vi "Pointer producer consumer TDMS generate file.vi"(7 "error in (no error)":errorcluster, 10 "Default Folder Path":string="c:\\Pointer_logs_raw\\") -> (0 "error out":errorcluster, 1 "channel name(s)":string[](array[string]), 2 "path":path, 3 "tdms file out":refnum<k34>)   [LabVIEW 2014]
panel:
  out "date/time string":string
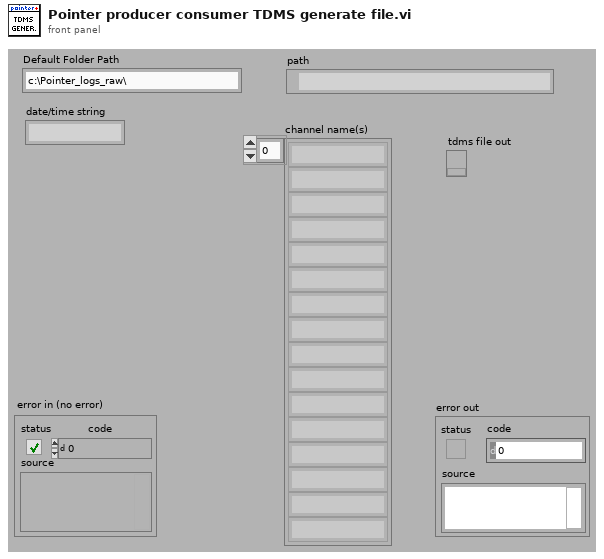
[diagram p1: front panel]
types:
  T1 = enum16{"open", "open or create", "create or replace", "create", "open (read-only)"}
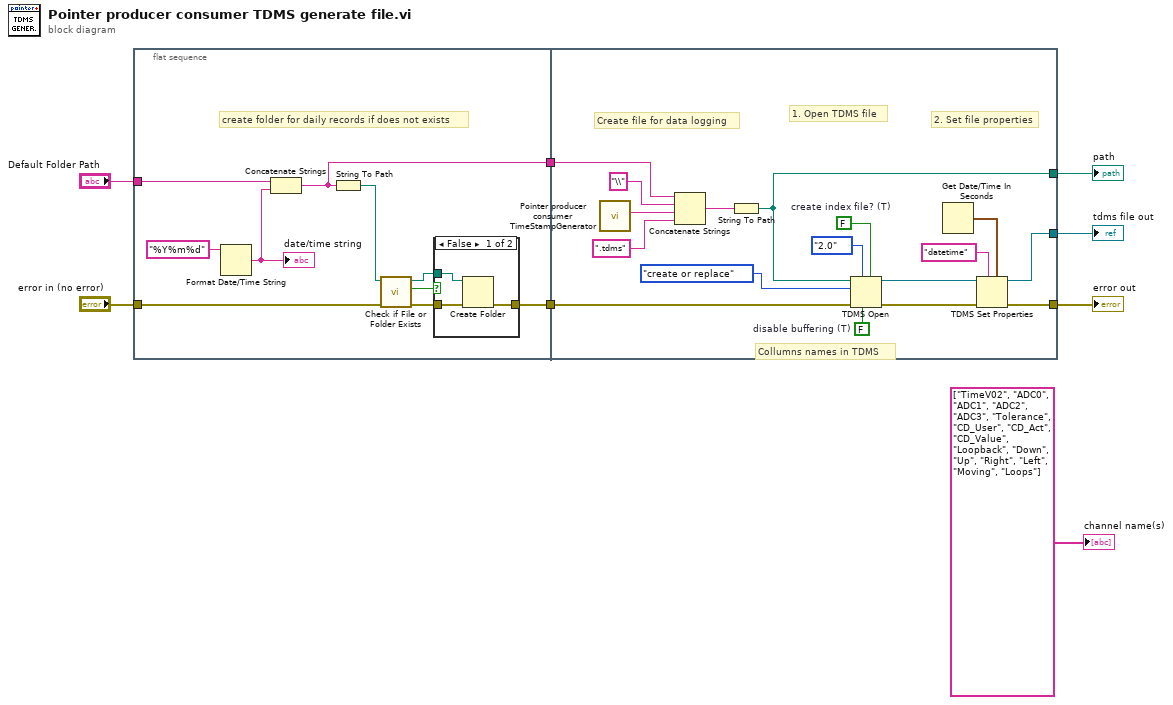
[diagram p0: block diagram]
diagram:
  # "Collumns names in TDMS"
  n1 = flat-sequence {
    tunnel: [w18] -> w8
    tunnel: "Default Folder Path" -> [w13]
    tunnel: [w10] -> w5
    tunnel: "error in (no error)" -> [w12]
    tunnel: w8 -> [w34]
    tunnel: w5 -> [w26]
    tunnel: [w25] -> w4
    tunnel: [w24] -> w3
    tunnel: [w23] -> w2
    frame #0 {
      # "create folder for daily records if does not exists"
      n2 = Format Date/Time String(time format string (%c)="%Y%m%d") -> (date/time string=w15:string)  [unwired: 2 in]
      "date/time string" <- w15
      n3 = Concatenate Strings(w13, w15) -> (w18:string)
      n4 = String To Path(string=w18) -> (path=w17:path)
      n5 = call <vilib>:"Check if File or Folder Exists.vi"("error in (no error)"=w12, "path"=w17) -> ("error out"=w11:errorcluster, "file or folder exists?"=w16:bool, "dup path"=w9:path)  [unwired: 7 in]
      n6 = case shown="False" w16 {
        tunnel: w11 -> [w21 w22]
        tunnel: [w20 w22] -> w10
        tunnel: w9 -> [w19 _]
        frame False {
          n7 = Create Folder(path (use dialog)=w19, error in=w21) -> (error out=w20:errorcluster)  [unwired: 1 in, 2 out]
        }
        frame True {
        }
      }
    }
    frame #1 {
      w27 = FALSE  # create index file? (T)
      w36 = FALSE  # disable buffering (T)
      # "Create file for data logging"
      # "2. Set file properties"
      # "1. Open TDMS file"
      n8 = call "Pointer producer consumer TimeStampGenerator.vi"() -> ("Local time (HHMMSS)"=w29:string)  [unwired: 8 in, 2 out]
      n9 = Concatenate Strings(w34, "\\" ("string"), w29, ".tdms") -> (w33:string)
      n10 = String To Path(string=w33) -> (path=w23:path)
      n11 = TDMS Open(5:w27, 6:w36, 7:enum16{"1.0", "2.0"}."2.0" ("file format version (2.0)"), 8:w26, 10:T1."create or replace" ("operation"), 11:w23) -> (0:w31:errorcluster, 3:w32:refnum<k34>)  [unwired: 1 in]
      n12 = Get Date/Time In Seconds() -> (seconds since 1Jan1904=w38:timestamp)
      n13 = TDMS Set Properties(5:w38, 7:"datetime", 8:w31, 11:w32) -> (0:w25:errorcluster, 3:w24:refnum<k34>)  [unwired: 4 out]
    }
  }
  "channel name(s)" <- string[] ["TimeV02", "ADC0", "ADC1", "ADC2", "ADC3", "Tolerance", "CD_User", "CD_Act", "CD_Value", "Loopback", "Down", "Up", "Right", "Left", "Moving", "Loops"] ("channel name(s) in (Untitled)")
  "error out" <- w4
  "tdms file out" <- w3
  "path" <- w2
